vi "ModifyGraph mirror.vi"(8 "error in (no error)":errorcluster, 10 "mirror [T]":bool=TRUE, 11 "ITX Commands in":refnum<class "ITX Commands.lvclass">) -> (0 "error out":errorcluster, 3 "ITX Commands out":refnum<class "ITX Commands.lvclass">)   [LabVIEW 2020, in "ITX Commands.lvclass"]
uses:
  ITX Commands.lvclass
  ITX Commands.lvclass/ITX Commands.ctl
panel:
  out "resulting string":string
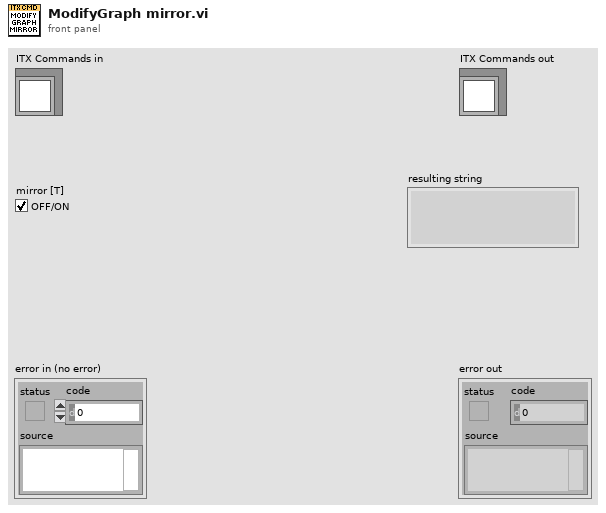
[diagram p1: front panel]
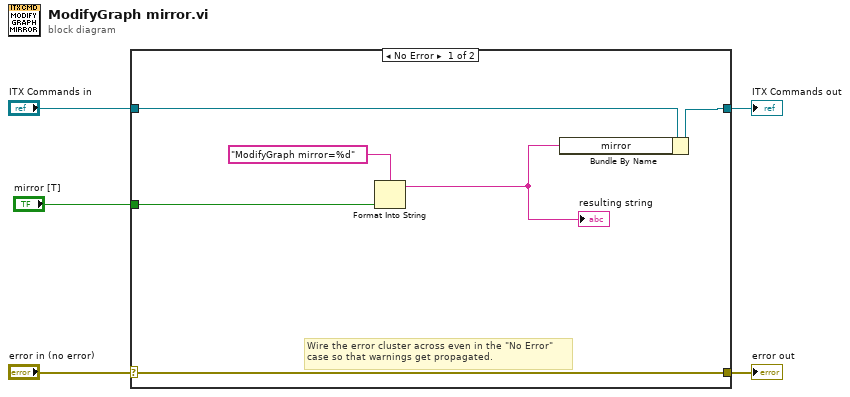
[diagram p0: block diagram]
diagram:
  n1 = case shown="No Error" "error in (no error)" {
    selector: "error in (no error)" -> [w11 w13]
    tunnel: [w11 w13] -> w4
    tunnel: [w9 w12] -> w2
    tunnel: "ITX Commands in" -> [w10 w12]
    tunnel: "mirror [T]" -> [w6 _]
    frame No Error {
      # "Wire the error cluster across even in the \"No Error\"\ncase so that warnings get propagated."
      n2 = Format Into String(format string="ModifyGraph mirror=%d", w6) -> (resulting string=w7:string)  [unwired: 2 in, 1 out]
      "resulting string" <- w7
      n3 = Bundle By Name(cluster=w10, "mirror"=w7) -> (w9:refnum<class "ITX Commands.lvclass">)
    }
    frame Error {
    }
  }
  "error out" <- w4
  "ITX Commands out" <- w2
